vi "CreatePublicEvents.vi"(8 "error in (no error)":errorcluster, 11 "Measurement":refnum<class "Measurement.lvclass">) -> (0 "error out":errorcluster, 3 "Measurement out":refnum<class "Measurement.lvclass">)   [LabVIEW 2017, in "Measurement.lvclass"]
doc: "JKI State Machine Objects (SMO) 1.3.0.56\nJKI - JKI\nCopyright (c) 2017, JKI"
uses:
  Measurement.lvclass
  Measurement.lvclass/Measurement.ctl
  Typedefs/PublicEvents--Measurement.Initialized.ctl
  Typedefs/Measurement.Measured--Data.ctl
  <vilib>/JKI/JKI SMO/SMO/SMO.lvclass
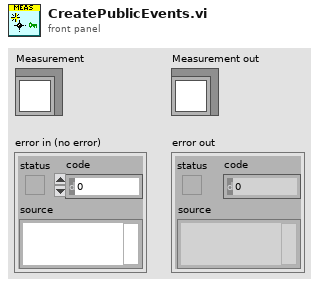
[diagram p1: front panel]
types:
  T1 = typedef "Measurement.lvclass/PrivateData--Ref.ctl" = refnum<data-value>
  T2 = typedef "Measurement.lvclass/Measurement.Measured--Data.ctl" = cluster{"Measurement Device":enum16{"SMU", "LIA", "OPM"}, "Result":variant}
  T3 = typedef "Measurement.lvclass/PublicEvents--Measurement.Initialized.ctl" = bool
  T4 = typedef "Measurement.lvclass/PrivateData--Cluster.ctl" = cluster{"Public Events":T5, "Protected Events":T6}
  T5 = typedef "Measurement.lvclass/PublicEvents--Cluster.ctl" = cluster{"Initialized":refnum<user-event>, "Measured":refnum<user-event>}
  T6 = typedef "Measurement.lvclass/ProtectedEvents--Cluster.ctl" = cluster{"Initialize":refnum<user-event>, "Begin":refnum<user-event>, "Pause":refnum<user-event>, "End":refnum<user-event>}
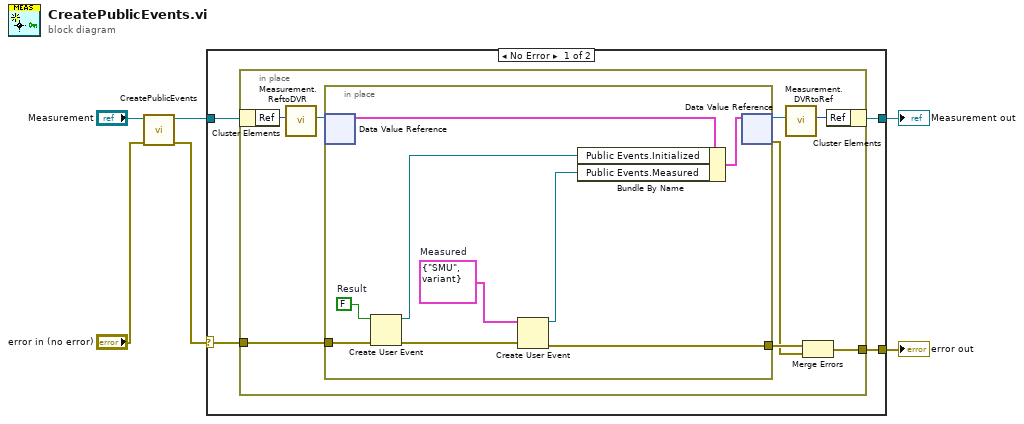
[diagram p0: block diagram]
diagram:
  n1 = call-parent "CreatePublicEvents.vi"("error in (no error)"="error in (no error)", "SMO"="Measurement") -> ("error out"=w3:errorcluster, "SMO out"=w4:refnum<class "Measurement.lvclass">)  [unwired: 8 in]
  n2 = case shown="No Error" w3 {
    selector: w3 -> [w9 w28]
    tunnel: w4 -> [w10 w29]
    tunnel: [w8 w28] -> w2
    tunnel: [w7 w29] -> w1
    frame No Error {
      n3 = in-place {
        in-place-border: w9 -> [w14]
        in-place-border: [w11] -> w8
        n4 = in-place-cluster #1(w10) -> ("Ref"=w18:u32)
        n5 = call "Measurement.ReftoDVR.vi"("Ref"=w18) -> ("Ref"=w17:T1)  [unwired: 10 in]
        n6 = in-place {
          in-place-border: w14 -> [w24]
          in-place-border: [w19] -> w13
          w20 = T2 {"Measurement Device"=enum."SMU", "Result"=variant}  # Measured
          w25 = T3 FALSE  # Result
          n7 = in-place-dvr #2(w17) -> (w27:T4)  [unwired: 1 out]
          n8 = Create User Event(user event datatype=w25, error in=w24) -> (user event=w23:refnum<user-event>, error out=w22:errorcluster)
          n9 = Create User Event(user event datatype=w20, error in=w22) -> (user event=w21:refnum<user-event>, error out=w19:errorcluster)
          n10 = Bundle By Name(cluster=w27, "Public Events.Initialized"=w23, "Public Events.Measured"=w21) -> (w26:T4)
          n11 = in-place-dvr #2(w26) -> (w16:T1, w12:errorcluster)
        }
        n12 = call "Measurement.DVRtoRef.vi"("Ref"=w16) -> ("Ref"=w15:u32)  [unwired: 10 in]
        n13 = Merge Errors(w13, w12) -> (w11:errorcluster)
        n14 = in-place-cluster #1("Ref"=w15) -> (w7:refnum<class "Measurement.lvclass">)
      }
    }
    frame Error {
    }
  }
  "error out" <- w2
  "Measurement out" <- w1
